vi "RectToCoordinates.vi"(0 "Rect":T3, 5 "Panel Origin":T1) -> (4 "Coordinates":T2)   [LabVIEW 2015, in "Front Panel Publisher.lvlib"]
uses:
  Front Panel Publisher.lvlib
  <vilib>/Utility/miscctls.llb/LVRectTypeDef.ctl
  Front Panel Objects/Object_class/Coordinates.ctl
  <vilib>/Utility/miscctls.llb/LVPointTypeDef.ctl
  Front Panel Objects/Object_class/Object.lvclass
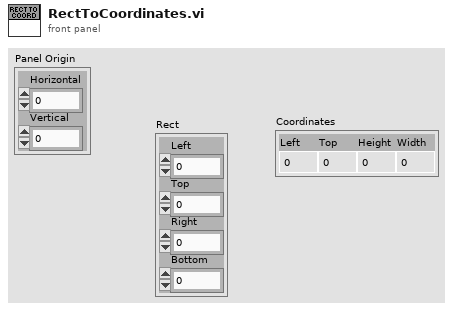
[diagram p1: front panel]
types:
  T1 = typedef "LVPointTypeDef.ctl" = cluster{"Horizontal":i16, "Vertical":i16}
  T2 = typedef "Front Panel Publisher.lvlib/Object.lvclass/Coordinates.ctl" = cluster{"Left":i32, "Top":i32, "Height":u32, "Width":u32}
  T3 = typedef "LVRectTypeDef.ctl" = cluster{"Left":i16, "Top":i16, "Right":i16, "Bottom":i16}
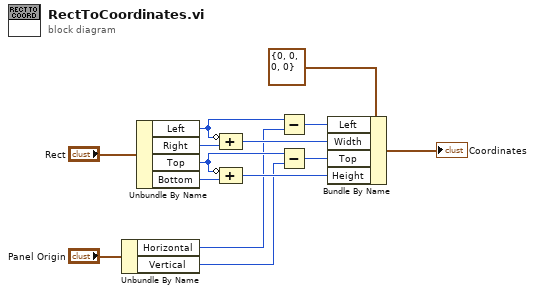
[diagram p0: block diagram]
diagram:
  n1 = Unbundle By Name("Panel Origin") -> ("Horizontal"=w3:i16, "Vertical"=w1:i16)
  n2 = Unbundle By Name("Rect") -> ("Left"=w11:i16, "Right"=w12:i16, "Top"=w8:i16, "Bottom"=w10:i16)
  n3 = Compound Arithmetic op=ADD(invert w11, w12) -> (w7:i16)
  n4 = Compound Arithmetic op=ADD(invert w8, w10) -> (w9:i16)
  n5 = Subtract(x=w11, y=w3) -> (x-y=w5:i16)
  n6 = Subtract(x=w8, y=w1) -> (x-y=w2:i16)
  n7 = Bundle By Name(cluster=T2 {"Left"=0, "Top"=0, "Height"=0, "Width"=0} ("Coordinates"), "Left"=w5, "Width"=w7, "Top"=w2, "Height"=w9) -> (→"Coordinates":T2)
